vi "Periodic Tasks.vi"(8 "error constant":errorcluster) -> ()   [LabVIEW 2019]
doc: "This VI runs in parallel to other tasks. It can contain as many user-defined periodic loops as you need. These can carry out PID or other sorts of timed response."
uses:
  <vilib>/Rock Robotics/WPI/ThirdParty/Phoenix-LabVIEW/Controls/CTRE_Phoenix_Params.ctl
  <vilib>/Rock Robotics/WPI/ThirdParty/Phoenix-LabVIEW/Motor Controller/Controls/CTRE_Phoenix_MotorControl_ControlMode.ctl
  <vilib>/Rock Robotics/WPI/ThirdParty/Phoenix-LabVIEW/Motor Controller/Controls/CTRE_Phoenix_MotorControl_MotionProfileControlMode.ctl
  <vilib>/Rock Robotics/WPI/Utilities/WPI_GetSetVariantRefNum.vi
  Constants.vi
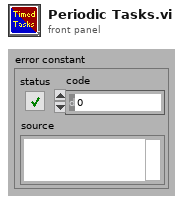
[diagram p1: front panel]
types:
  T1 = enum16{"One_Axis_PercentOutput", "Two_Axis_PercentOutput", "One_Axix_Position", "One_Axis_Position_CustomFeedFwd", "Two_Axis_Position", "One_Axis_Velocity", "One_Axis_Velocity_CustomFeedFwd", "Two_Axis_Velocity", "One_Axis_MotionMagic", "One_Axis_MotionMagic_CustomFeedFwd", "Two_Axis_MotionMagic", "One_Axis_MotionProfile", "One_Axis_MotionProfile_CustomFeedFwd", "Two_Axis_MotionProfile", "Two_Axis_MotionProfile_CustomFeedFwd"}
  T2 = typedef "WPI_MotorControlDeviceRef.ctl" = cluster{"DeviceStatus":errorcluster, "Type":T3, "PWM":cluster{"PWM Channel":T4, "DeadBand":T5}, "CAN":cluster{"Device Number":u8, "SetOutput VI Ref":variant, "GetOutput VI Ref":variant, "Enable VI Ref":variant, "Disable VI Ref":variant, "Data":variant}, "Invert":bool, "DIO PWM":cluster{"PWM \"Enable\" Channel":T4, "DIOChannel":T6, "PWM Rate":dbl}}
  T3 = typedef "WPI_MotorControlType.ctl" = enum16{"PWM", "CAN", "DIO PWM"}
  T4 = typedef "FPGA_DIOPWMChannel.ctl" = enum8{"PWM 0", "PWM 1", "PWM 2", "PWM 3", "PWM 4", "PWM 5", "PWM 6", "PWM 7", "PWM 8", "PWM 9", "PWM MXP 0", "PWM MXP 1", "PWM MXP 2", "PWM MXP 3", "PWM MXP 4", "PWM MXP 5", "PWM MXP 6", "PWM MXP 7", "PWM MXP 8", "PWM MXP 9", "Invalid"}
  T5 = typedef "WPI_PWMDeadband.ctl" = cluster{"Name":string, "maxPositivePwm":i32, "minPositivePwm":i32, "centerPwm":i32, "maxNegativePwm":i32, "minNegativePwm":i32, "angularRange":u16}
  T6 = typedef "FPGA_DIOChannel.ctl" = enum8{"DIO 0", "DIO 1", "DIO 2", "DIO 3", "DIO 4", "DIO 5", "DIO 6", "DIO 7", "DIO 8", "DIO 9", "DIO MXP 0", "DIO MXP 1", "DIO MXP 2", "DIO MXP 3", "DIO MXP 4", "DIO MXP 5", "DIO MXP 6", "DIO MXP 7", "DIO MXP 8", "DIO MXP 9", "DIO MXP 10", "DIO MXP 11", "DIO MXP 12", "DIO MXP 13", "DIO MXP 14", "DIO MXP 15", "SPI Port CS1", "SPI Port CS2", "SPI Port CS3", "SPI Port MISO", "SPI Port MOSI", "Invalid"}
  T7 = typedef "CTRE_PigeonIMU_DeviceRef.ctl" = cluster{"DeviceStatus":errorcluster, "Device Number":u8, "Type":T8, "Device ID":u32, "Handle":u64, "UsageFrame":u32, "Library Path":path}
  T8 = typedef "CTRE_PigeonIMU_ConnectionType.ctl" = u32
  T9 = typedef "WPI_JoystickDevRef.ctl" = cluster{"Device":T10}
  T10 = typedef "WPI_JoystickDeviceEnum.ctl" = enum16{"USB 0", "USB 1", "USB 2", "USB 3", "USB 4", "USB 5"}
  T11 = enum16{"DemandType_Neutral", "DemandType_AuxPID", "DemandType_ArbitraryFeedForward"}
  T12 = enum16{"FollowerType_PercentOutput", "FollowerType_AuxOutput1"}
  T13 = enum16{"One_Axis_PercentOutput", "Two_Axis_PercentOutput", "One_Axix_Position", "One_Axis_Position_CustomFeedFwd", "Two_Axis_Position", "One_Axis_Velocity", "One_Axis_Velocity_CustomFeedFwd", "Two_Axis_Velocity", "One_Axis_MotionMagic", "One_Axis_MotionMagic_CustomFeedFwd", "Two_Axis_MotionMagic", "One_Axis_MotionProfile", "Two_Axis_MotionProfile"}
  T14 = typedef "CTRE_Phoenix_Params.ctl" = u16
  T15 = typedef "CTRE_Phoenix_MotorControl_ControlMode.ctl" = u16
  T16 = typedef "CTRE_Phoenix_MotorControl_MotionProfileControlMode.ctl" = u16
  T17 = typedef "CTRE_Phoenix_MotorControl_BufferedTrajectoryPointStream_DeviceRef.ctl" = cluster{"Handle":u64, "Library Path":path}
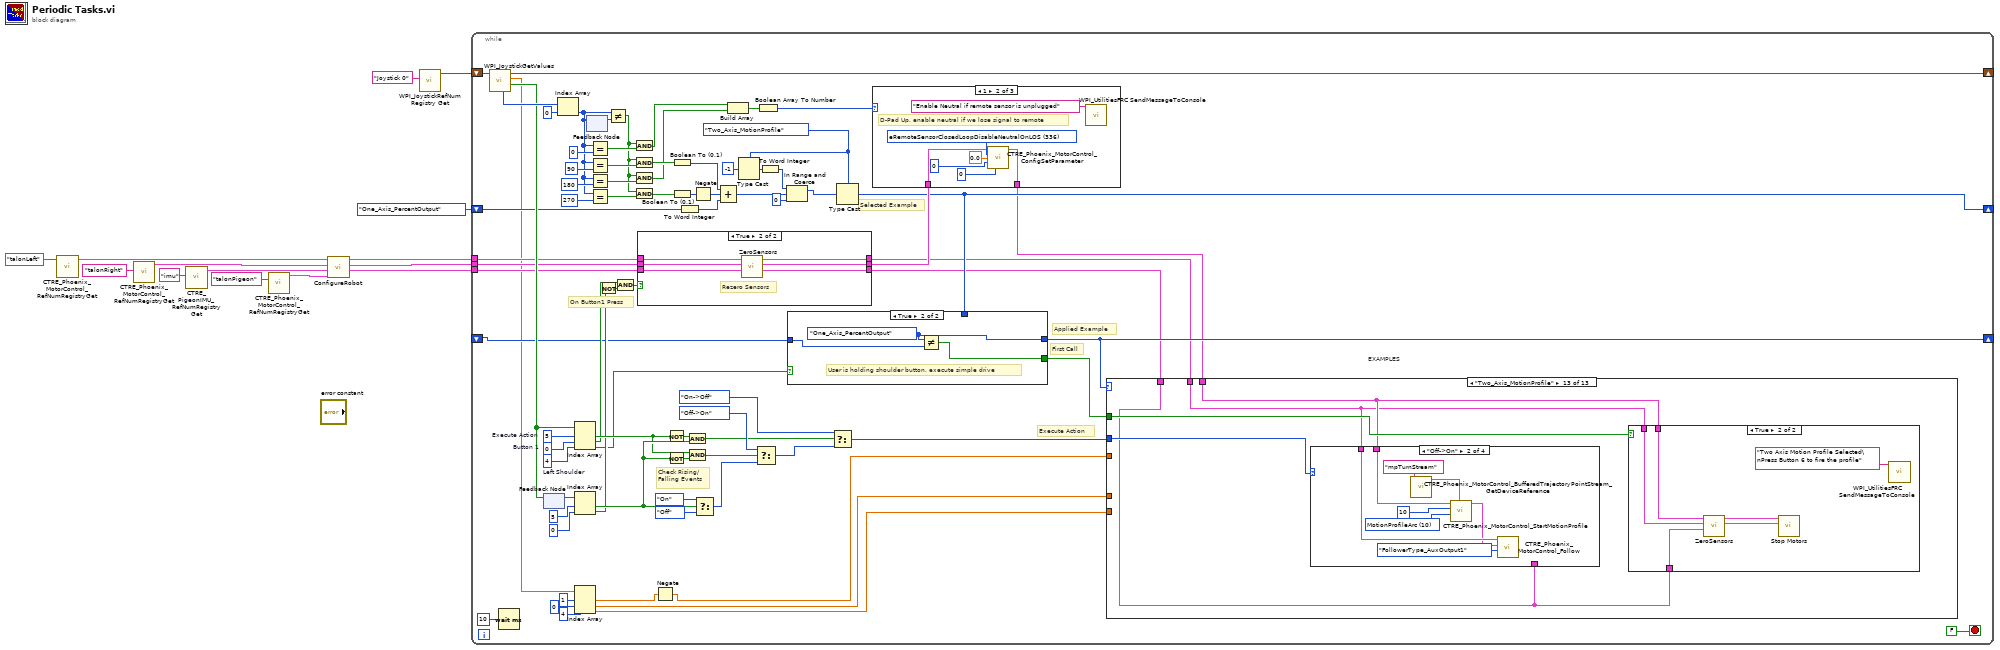
[diagram p0: block diagram]
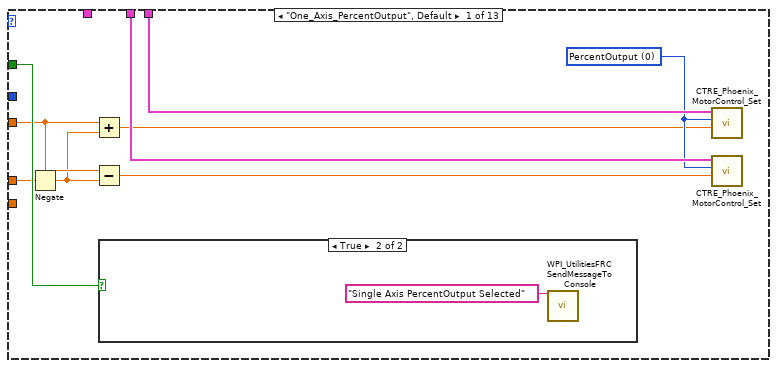
[diagram p2: hidden frame]
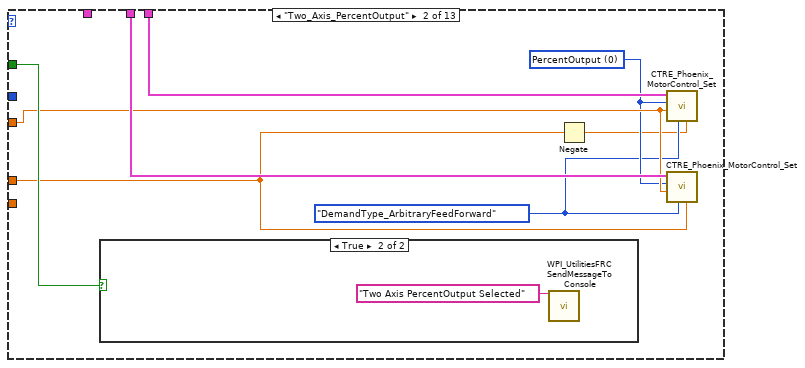
[diagram p4: hidden frame]
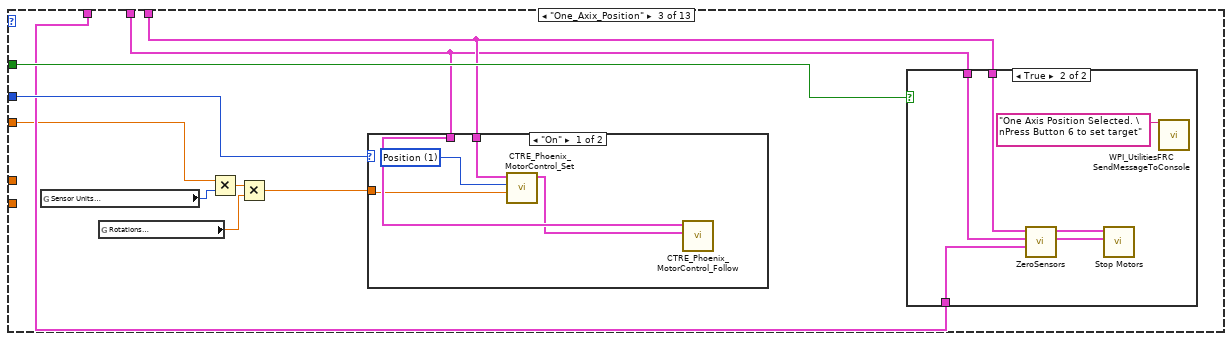
[diagram p6: hidden frame]
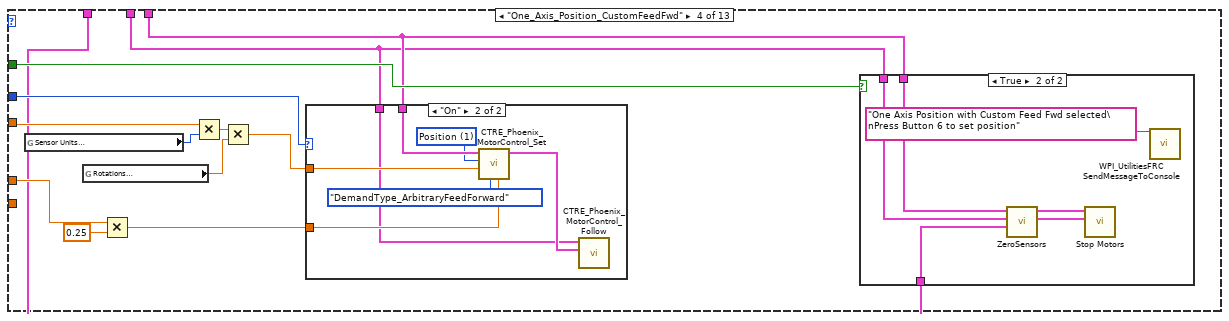
[diagram p9: hidden frame]
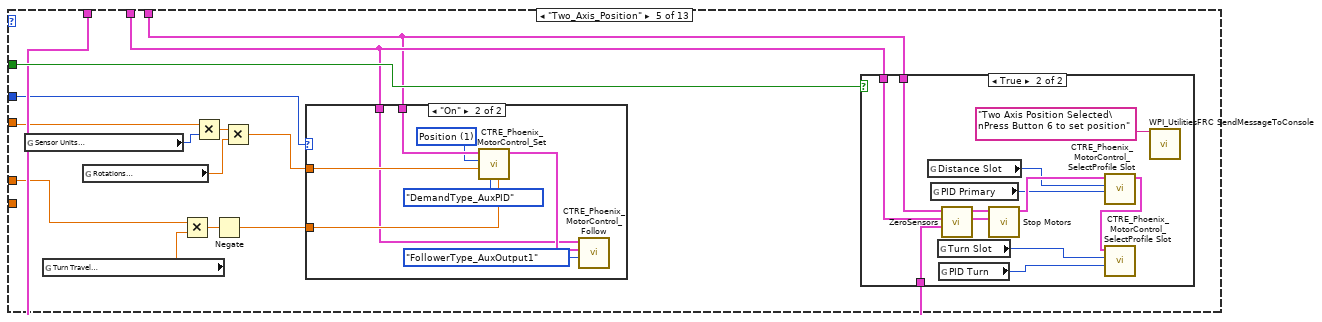
[diagram p12: hidden frame]
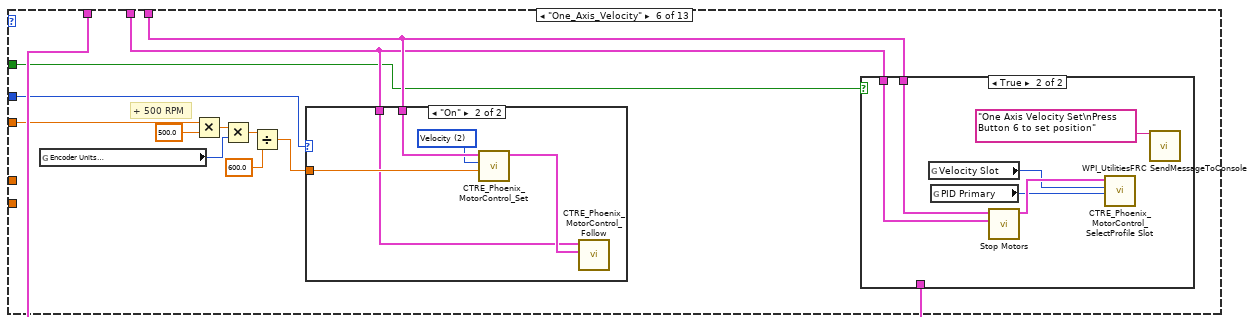
[diagram p15: hidden frame]
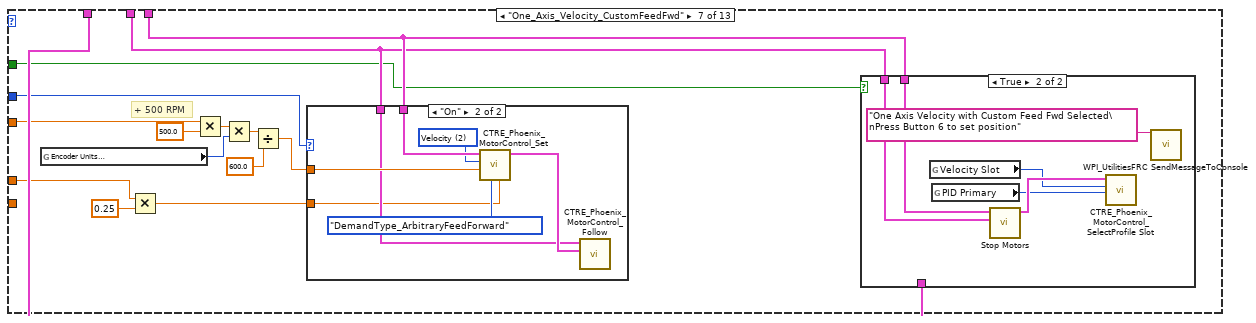
[diagram p18: hidden frame]
diagram:
  n1 = call <vilib>:"CTRE_Phoenix_MotorControl_RefNumRegistryGet.vi"("refnum name"="talonLeft") -> ("PhoenixMotorControlDevRef"=w7:T2)  [unwired: 9 in, 1 out]
  n2 = call <vilib>:"CTRE_Phoenix_MotorControl_RefNumRegistryGet.vi"("refnum name"="talonRight") -> ("PhoenixMotorControlDevRef"=w8:T2)  [unwired: 9 in, 1 out]
  n3 = call <vilib>:"CTRE_PigeonIMU_RefNumRegistryGet.vi"("refnum name"="imu") -> ("PigeonIMUDevRef"=w3:T7)  [unwired: 9 in, 1 out]
  n4 = call <vilib>:"CTRE_Phoenix_MotorControl_RefNumRegistryGet.vi"("refnum name"="talonPigeon") -> ("PhoenixMotorControlDevRef"=w2:T2)  [unwired: 9 in, 1 out]
  n5 = call "ConfigureRobot.vi"("Pigeon Talon"=w2, "Pigeon"=w3, "Right Side"=w8, "Left Side"=w7) -> ("Pigeon 2"=w4:T7, "Right Side 2"=w1:T2, "Left Side 2"=w5:T2)  [unwired: 5 in]
  n6 = call <vilib>:"WPI_JoystickRefNum Registry Get.vi"("refnum name"="Joystick 0") -> ("JoystickDevRef"=w13:T9)  [unwired: 1 in, 9 out]
  n7 = while {
    shift-right: [w90] -> _
    shift-left: w13 -> [w91]
    shift-right: [w40] -> _
    shift-left: T1."One_Axis_PercentOutput" -> [w39]
    tunnel: w5 -> [w54]
    tunnel: w1 -> [w53]
    tunnel: w4 -> [w52]
    shift-right: [w41] -> _
    shift-left: _ -> [w42]
    stop <- FALSE stop-if-true
    w33 = T13."Two_Axis_MotionProfile"
    w44 = 4  # Left Shoulder
    w50 = 0  # Button 1
    w68 = 5  # Execute Action
    # "Execute Action"
    # "Check Rising/\nFalling Events"
    # "First Call"
    # "Applied Example"
    # "On Button1 Press"
    # "Selected Example"
    n8 = call <vilib>:"WPI_JoystickGetValues.vi"("JoystickDevRef"=w91) -> ("Buttons"=w70:bool[], "Axes"=w28:dbl[], "JoystickDevRef"=w90:T9, "POVs"=w89:i16[])  [unwired: 6 in, 1 out]
    n9 = Wait (ms)(milliseconds to wait=u32 10) -> ()  [unwired: 1 out]
    n10 = feedback #1() -> (w69:bool[])  [unwired: 1 in]
    n11 = feedback-in #1(w70) -> ()
    n12 = Index Array(array=w89, index=0) -> (element=w82:i16)
    n13 = Index Array(array=w70, index #1=w68, index #2=w50, index #3=w44) -> (element #1=w61:bool, element #2=w47:bool, element #3=w43:bool)
    n14 = Index Array(array=w69, index #1=5 ("index"), index #2=0 ("index")) -> (element #1=w62:bool, element #2=w45:bool)
    n15 = Index Array(array=w28, index #1=1 ("index"), index #2=0 ("index"), index #3=4 ("index")) -> (element #1=w17:dbl, element #2=w25:dbl, element #3=w18:dbl)
    n16 = feedback #2() -> (w83:i16)  [unwired: 1 in]
    n17 = feedback-in #2(w82) -> ()
    n18 = Equal?(x=w82, y=i16 0) -> (x = y?=w81:bool)
    n19 = Equal?(x=w82, y=i16 90) -> (x = y?=w80:bool)
    n20 = Equal?(x=w82, y=i16 180) -> (x = y?=w79:bool)
    n21 = Equal?(x=w82, y=i16 270) -> (x = y?=w78:bool)
    n22 = Not(x=w45) -> (.not. x?=w46:bool)
    n23 = Not Equal?(x=w82, y=w83) -> (x != y?=w77:bool)
    n24 = And(x=w47, y=w46) -> (x .and. y?=w48:bool)
    n25 = And(x=w77, y=w81) -> (x .and. y?=w72:bool)
    n26 = And(x=w77, y=w80) -> (x .and. y?=w75:bool)
    n27 = And(x=w77, y=w79) -> (x .and. y?=w71:bool)
    n28 = And(x=w77, y=w78) -> (x .and. y?=w76:bool)
    n29 = case shown="True" w48 {
      tunnel: w54 -> [w422 w424]
      tunnel: w53 -> [w423 w425]
      tunnel: w52 -> [w421 w426]
      tunnel: [w423 w428] -> w51
      tunnel: [w422 w429] -> w24
      tunnel: [w421 w427] -> w15
      frame False {
        # "Do Nothing"
      }
      frame True {
        # "Rezero Sensors"
        n30 = call "ZeroSensors.vi"("Pigeon"=w426, "Talon 2"=w425, "Talon 1"=w424) -> ("Pigeon"=w427:T7, "Talon 2"=w428:T2, "Talon 1"=w429:T2)  [unwired: 6 in]
      }
    }
    n31 = Negate(x=w17) -> (-x=w16:dbl)
    n32 = Not(x=w61) -> (.not. x?=w63:bool)
    n33 = Not(x=w62) -> (.not. x?=w64:bool)
    n34 = Boolean To (0,1)(Boolean=w75) -> (0, 1=w22:i16)
    n35 = Boolean To (0,1)(Boolean=w76) -> (0, 1=w20:i16)
    n36 = To Word Integer(number=w39) -> (16bit integer=w38:i16)
    n37 = And(x=w63, y=w62) -> (x .and. y?=w55:bool)
    n38 = And(x=w61, y=w64) -> (x .and. y?=w56:bool)
    n39 = Negate(x=w20) -> (-x=w21:i16)
    n40 = Select(t=enum16{"Off->On", "On->Off", "On", "Off"}."On", s=w62, f=enum16{"Off->On", "On->Off", "On", "Off"}."Off") -> (s? t:f=w60:enum16{"Off->On", "On->Off", "On", "Off"})
    n41 = Compound Arithmetic op=ADD(w22, w21, w38) -> (w37:i16)
    n42 = Build Array(w72, w71) -> (w73:bool[])
    n43 = Type Cast(type=w33, x=i16 -1 ("lower limit")) -> (*(type *) &x=w31:T13)
    n44 = Select(t=enum16{"Off->On", "On->Off", "On", "Off"}."Off->On", s=w56, f=w60) -> (s? t:f=w59:enum16{"Off->On", "On->Off", "On", "Off"})
    n45 = Boolean Array To Number(Boolean array=w73) -> (number=w74:u32)
    n46 = To Word Integer(number=w31) -> (16bit integer=w32:i16)
    n47 = In Range and Coerce(upper limit=w32, x=w37, lower limit=i16 0) -> (coerced(x)=w35:i16)  [unwired: 1 out]
    n48 = Select(t=enum16{"Off->On", "On->Off", "On", "Off"}."On->Off", s=w55, f=w59) -> (s? t:f=w29:enum16{"Off->On", "On->Off", "On", "Off"})
    n49 = Type Cast(type=w33, x=w35) -> (*(type *) &x=w40:T13)
    n50 = case shown="True" w43 {
      tunnel: w42 -> [w415 w420]
      tunnel: [w417 w419] -> w30
      tunnel: [w416 w418] -> w41
      tunnel: w40 -> [w416 _]
      frame False {
        # "User is not holding shoulder button, use applied example"
        n51 = Not Equal?(x=w416, y=w415) -> (x != y?=w417:bool)
      }
      frame True {
        w418 = T13."One_Axis_PercentOutput"
        # "User is holding shoulder button, execute simple drive"
        n52 = Not Equal?(x=w418, y=w420) -> (x != y?=w419:bool)
      }
    }
    n53 = case shown="1" w74 {
      tunnel: w51 -> [w430 w432 w444]
      tunnel: [w430 w433 w443] -> w23
      frame 0, Default {
        # "Nothing Pressed"
      }
      frame 1 {
        w437 = T14 336 items=["eOnBoot_BrakeMode"=31, "eQuadFilterEn"=91, "eQuadIdxPolarity"=108, "eClearPositionOnIdx"=100, "eMotionProfileHasUnderrunErr"=119, "eMotionProfileTrajectoryPointDurationMs"=120, "eClearPosOnLimitF"=144, "eClearPosOnLimitR"=145, "eStatusFramePeriod"=300, "eOpenLoopRamp"=301, "eClosedLoopRamp"=302, "eNeutralDeadband"=303, "ePeakPosOutput"=305, "eNominalPosOutput"=306, "ePeakNegOutput"=307, "eNominalNegOutput"=308, "eProfileParamSlot_P"=310, "eProfileParamSlot_I"=311, "eProfileParamSlot_D"=312, "eProfileParamSlot_F"=313, "eProfileParamSlot_IZone"=314, "eProfileParamSlot_AllowableErr"=315, "eProfileParamSlot_MaxIAccum"=316, "eClearPositionOnLimitF"=320, "eClearPositionOnLimitR"=321, "eClearPositionOnQuadIdx"=322, "eSampleVelocityPeriod"=325, "eSampleVelocityWindow"=326, "eFeedbackSensorType"=330, "eSelectedSensorPosition"=331, "eFeedbackNotContinuous"=332, "eRemoteSensorSource"=333, "eRemoteSensorDeviceID"=334, "eSensorTerm"=335, "eRemoteSensorClosedLoopDisableNeutralOnLOS"=336, "eForwardSoftLimitThreshold"=340, "eReverseSoftLimitThreshold"=341, "eForwardSoftLimitEnable"=342, "eReverseSoftLimitEnable"=343, "eNominalBatteryVoltage"=350, "eBatterVoltageFilterSize"=351, "eContinuousCurrentLimitAmps"=360, "eContinuousCurrentLimitMs"=361, "ePeakCurrentLimitAmps"=362, "eClosedLoopIAccum"=370, "eCustomParam"=380, "eStickyFaults"=390, "eAnalogPosition"=400, "eQuadraturePosition"=401, "ePulseWidthPosition"=402, "eMotMag_Accel"=410, "eMotMag_VelCruise"=411, "eLimitSwitchSource"=421, "eLimitSwitchNormClosedAndDis"=422, "eLimitSwitchDisabledNeutralOnLOS"=423, "eLimitSwitchRemoteDevID"=424] ("Parameter")
        # "D-Pad Up, enable neutral if we lose signal to remote"
        n54 = call <vilib>:"CTRE_Phoenix_MotorControl_ConfigSetParameter.vi"("PhoenixMotorControlDevRef"=w432, "Parameter"=w437, "value"=0.0, "subValue"=u8 0, "ordinal"=0) -> ("PhoenixMotorControlDevRef"=w433:T2)  [unwired: 9 in, 1 out]
        n55 = call <vilib>:"WPI_UtilitiesFRC SendMessageToConsole.vi"("Message"="Enable Neutral if remote sensor is unplugged") -> ()  [unwired: 14 in, 1 out]
      }
      frame 2 {
        w442 = T14 336 items=["eOnBoot_BrakeMode"=31, "eQuadFilterEn"=91, "eQuadIdxPolarity"=108, "eClearPositionOnIdx"=100, "eMotionProfileHasUnderrunErr"=119, "eMotionProfileTrajectoryPointDurationMs"=120, "eClearPosOnLimitF"=144, "eClearPosOnLimitR"=145, "eStatusFramePeriod"=300, "eOpenLoopRamp"=301, "eClosedLoopRamp"=302, "eNeutralDeadband"=303, "ePeakPosOutput"=305, "eNominalPosOutput"=306, "ePeakNegOutput"=307, "eNominalNegOutput"=308, "eProfileParamSlot_P"=310, "eProfileParamSlot_I"=311, "eProfileParamSlot_D"=312, "eProfileParamSlot_F"=313, "eProfileParamSlot_IZone"=314, "eProfileParamSlot_AllowableErr"=315, "eProfileParamSlot_MaxIAccum"=316, "eClearPositionOnLimitF"=320, "eClearPositionOnLimitR"=321, "eClearPositionOnQuadIdx"=322, "eSampleVelocityPeriod"=325, "eSampleVelocityWindow"=326, "eFeedbackSensorType"=330, "eSelectedSensorPosition"=331, "eFeedbackNotContinuous"=332, "eRemoteSensorSource"=333, "eRemoteSensorDeviceID"=334, "eSensorTerm"=335, "eRemoteSensorClosedLoopDisableNeutralOnLOS"=336, "eForwardSoftLimitThreshold"=340, "eReverseSoftLimitThreshold"=341, "eForwardSoftLimitEnable"=342, "eReverseSoftLimitEnable"=343, "eNominalBatteryVoltage"=350, "eBatterVoltageFilterSize"=351, "eContinuousCurrentLimitAmps"=360, "eContinuousCurrentLimitMs"=361, "ePeakCurrentLimitAmps"=362, "eClosedLoopIAccum"=370, "eCustomParam"=380, "eStickyFaults"=390, "eAnalogPosition"=400, "eQuadraturePosition"=401, "ePulseWidthPosition"=402, "eMotMag_Accel"=410, "eMotMag_VelCruise"=411, "eLimitSwitchSource"=421, "eLimitSwitchNormClosedAndDis"=422, "eLimitSwitchDisabledNeutralOnLOS"=423, "eLimitSwitchRemoteDevID"=424] ("Parameter")
        # "D-Pad Up, disable neutral if we lose signal to remote"
        n56 = call <vilib>:"CTRE_Phoenix_MotorControl_ConfigSetParameter.vi"("PhoenixMotorControlDevRef"=w444, "Parameter"=w442, "value"=1.0, "subValue"=u8 0, "ordinal"=0) -> ("PhoenixMotorControlDevRef"=w443:T2)  [unwired: 9 in, 1 out]
        n57 = call <vilib>:"WPI_UtilitiesFRC SendMessageToConsole.vi"("Message"="Disable Neutral if remote sensor is unplugged") -> ()  [unwired: 14 in, 1 out]
      }
    }
    n58 = case "EXAMPLES" shown="\"Two_Axis_MotionProfile\"" w41 {
      tunnel: w30 -> [w100 w111 w122 w146 w169 w201 w222 w254 w282 w308 w328 w364 w392]
      tunnel: w29 -> [_ _ w121 w145 w165 w200 w221 w253 w281 w309 w334 w363 w391]
      tunnel: w16 -> [w98 w108 w113 w141 w164 w199 w220 w252 w280 w310 w333 _ _]
      tunnel: w25 -> [w95 w105 _ w140 w163 _ w219 w251 _ w304 w332 _ _]
      tunnel: w24 -> [w101 w109 w115 w135 w167 w203 w224 w249 w283 w306 w330 w365 w389]
      tunnel: w23 -> [w102 w110 w116 w136 w166 w204 w225 w248 w285 w305 w329 w366 w390]
      tunnel: w15 -> [_ _ w114 w134 w168 w202 w223 w250 w284 w307 w331 w362 w388]
      tunnel: w18 -> [_ _ _ _ _ _ _ _ _ _ _ _ _]
      frame "One_Axis_PercentOutput", Default {
        w99 = T15 0 items=["PercentOutput"=0, "Position"=1, "Velocity"=2, "Current"=3, "Follower"=5, "MotionProfile"=6, "MotionMagic"=7, "MotionMagicArc"=8, "MotionProfileArc"=10, "Disabled"=15] ("Control Mode")
        n59 = Negate(x=w95) -> (-x=w94:dbl)
        n60 = Add(x=w98, y=w94) -> (x+y=w96:dbl)
        n61 = Subtract(x=w98, y=w94) -> (x-y=w97:dbl)
        n62 = case shown="True" w100 {
          frame False {
          }
          frame True {
            n63 = call <vilib>:"WPI_UtilitiesFRC SendMessageToConsole.vi"("Message"="Single Axis PercentOutput Selected") -> ()  [unwired: 14 in, 1 out]
          }
        }
        n64 = call <vilib>:"CTRE_Phoenix_MotorControl_Set.vi"("Output"=w96, "Control Mode"=w99, "PhoenixMotorControlDevRef"=w102) -> ()  [unwired: 7 in, 2 out]
        n65 = call <vilib>:"CTRE_Phoenix_MotorControl_Set.vi"("Output"=w97, "Control Mode"=w99, "PhoenixMotorControlDevRef"=w101) -> ()  [unwired: 7 in, 2 out]
      }
      frame "Two_Axis_PercentOutput" {
        w106 = T11."DemandType_ArbitraryFeedForward" ("DemandType")
        w107 = T15 0 items=["PercentOutput"=0, "Position"=1, "Velocity"=2, "Current"=3, "Follower"=5, "MotionProfile"=6, "MotionMagic"=7, "MotionMagicArc"=8, "MotionProfileArc"=10, "Disabled"=15] ("Control Mode")
        n66 = case shown="True" w111 {
          frame False {
          }
          frame True {
            n67 = call <vilib>:"WPI_UtilitiesFRC SendMessageToConsole.vi"("Message"="Two Axis PercentOutput Selected") -> ()  [unwired: 14 in, 1 out]
          }
        }
        n68 = Negate(x=w105) -> (-x=w104:dbl)
        n69 = call <vilib>:"CTRE_Phoenix_MotorControl_Set.vi"("Demand1"=w104, "DemandType"=w106, "Output"=w108, "Control Mode"=w107, "PhoenixMotorControlDevRef"=w110) -> ()  [unwired: 5 in, 2 out]
        n70 = call <vilib>:"CTRE_Phoenix_MotorControl_Set.vi"("Demand1"=w105, "DemandType"=w106, "Output"=w108, "Control Mode"=w107, "PhoenixMotorControlDevRef"=w109) -> ()  [unwired: 5 in, 2 out]
      }
      frame "One_Axix_Position" {
        n71 = global read "Constants.vi" "Sensor Units\nPer Rotation"() -> (w119:i32)
        n72 = global read "Constants.vi" "Rotations\nTo Travel"() -> (w118:dbl)
        n73 = Multiply(x=w113, y=w119) -> (x*y=w120:dbl)
        n74 = Multiply(x=w120, y=w118) -> (x*y=w117:dbl)
        n75 = case shown="\"On\"" w121 {
          tunnel: w117 -> [w123 _]
          tunnel: w116 -> [w127 _]
          tunnel: w115 -> [w125 _]
          frame "On" {
            w126 = T15 1 items=["PercentOutput"=0, "Position"=1, "Velocity"=2, "Current"=3, "Follower"=5, "MotionProfile"=6, "MotionMagic"=7, "MotionProfileArc"=10, "Disabled"=15] ("Control Mode")
            n76 = call <vilib>:"CTRE_Phoenix_MotorControl_Set.vi"("Output"=w123, "Control Mode"=w126, "PhoenixMotorControlDevRef"=w127) -> ("PhoenixMotorControlDevRef"=w124:T2)  [unwired: 7 in, 1 out]
            n77 = call <vilib>:"CTRE_Phoenix_MotorControl_Follow.vi"("Master Controller to Follow"=w124, "PhoenixMotorControlDevRef"=w125) -> ()  [unwired: 8 in, 2 out]
          }
          frame Default {
          }
        }
        n78 = case shown="True" w122 {
          tunnel: w116 -> [_ w132]
          tunnel: w115 -> [_ w131]
          tunnel: w114 -> [_ w130]
          frame False {
          }
          frame True {
            n79 = call "ZeroSensors.vi"("Pigeon"=w130, "Talon 2"=w131, "Talon 1"=w132) -> ("Talon 2"=w128:T2, "Talon 1"=w129:T2)  [unwired: 6 in, 1 out]
            n80 = call "Stop Motors.vi"("Talon SRX 2"=w128, "Talon SRX 1"=w129) -> ()  [unwired: 8 in, 2 out]
            n81 = call <vilib>:"WPI_UtilitiesFRC SendMessageToConsole.vi"("Message"="One Axis Position Selected. \nPress Button 6 to set target") -> ()  [unwired: 14 in, 1 out]
          }
        }
      }
      frame "One_Axis_Position_CustomFeedFwd" {
        n82 = global read "Constants.vi" "Sensor Units\nPer Rotation"() -> (w143:i32)
        n83 = global read "Constants.vi" "Rotations\nTo Travel"() -> (w142:dbl)
        n84 = Multiply(x=w140, y=0.25) -> (x*y=w137:dbl)
        n85 = Multiply(x=w141, y=w143) -> (x*y=w144:dbl)
        n86 = Multiply(x=w144, y=w142) -> (x*y=w138:dbl)
        n87 = case shown="\"On\"" w145 {
          tunnel: w136 -> [_ w153]
          tunnel: w135 -> [_ w147]
          tunnel: w137 -> [_ w149]
          tunnel: w138 -> [_ w151]
          frame Default {
          }
          frame "On" {
            w152 = T15 1 items=["PercentOutput"=0, "Position"=1, "Velocity"=2, "Current"=3, "Follower"=5, "MotionProfile"=6, "MotionMagic"=7, "MotionProfileArc"=10, "Disabled"=15] ("Control Mode")
            n88 = call <vilib>:"CTRE_Phoenix_MotorControl_Set.vi"("Demand1"=w149, "DemandType"=T11."DemandType_ArbitraryFeedForward", "Output"=w151, "Control Mode"=w152, "PhoenixMotorControlDevRef"=w153) -> ("PhoenixMotorControlDevRef"=w148:T2)  [unwired: 5 in, 1 out]
            n89 = call <vilib>:"CTRE_Phoenix_MotorControl_Follow.vi"("Master Controller to Follow"=w148, "PhoenixMotorControlDevRef"=w147) -> ()  [unwired: 8 in, 2 out]
          }
        }
        n90 = case shown="True" w146 {
          tunnel: w136 -> [_ w156]
          tunnel: w135 -> [_ w155]
          tunnel: w134 -> [_ w154]
          frame False {
          }
          frame True {
            n91 = call "ZeroSensors.vi"("Pigeon"=w154, "Talon 2"=w155, "Talon 1"=w156) -> ("Talon 2"=w157:T2, "Talon 1"=w158:T2)  [unwired: 6 in, 1 out]
            n92 = call "Stop Motors.vi"("Talon SRX 2"=w157, "Talon SRX 1"=w158) -> ()  [unwired: 8 in, 2 out]
            n93 = call <vilib>:"WPI_UtilitiesFRC SendMessageToConsole.vi"("Message"="One Axis Position with Custom Feed Fwd selected\nPress Button 6 to set position") -> ()  [unwired: 14 in, 1 out]
          }
        }
      }
      frame "Two_Axis_Position" {
        n94 = global read "Constants.vi" "Sensor Units\nPer Rotation"() -> (w172:i32)
        n95 = global read "Constants.vi" "Turn Travel\nUnits Per Rotation"() -> (w162:dbl)
        n96 = global read "Constants.vi" "Rotations\nTo Travel"() -> (w171:dbl)
        n97 = Multiply(x=w163, y=w162) -> (x*y=w161:dbl)
        n98 = Multiply(x=w164, y=w172) -> (x*y=w173:dbl)
        n99 = Negate(x=w161) -> (-x=w160:dbl)
        n100 = Multiply(x=w173, y=w171) -> (x*y=w170:dbl)
        n101 = case shown="\"On\"" w165 {
          tunnel: w166 -> [_ w181]
          tunnel: w167 -> [_ w175]
          tunnel: w160 -> [_ w177]
          tunnel: w170 -> [_ w179]
          frame Default {
          }
          frame "On" {
            w180 = T15 1 items=["PercentOutput"=0, "Position"=1, "Velocity"=2, "Current"=3, "Follower"=5, "MotionProfile"=6, "MotionMagic"=7, "MotionProfileArc"=10, "Disabled"=15] ("Control Mode")
            n102 = call <vilib>:"CTRE_Phoenix_MotorControl_Set.vi"("Demand1"=w177, "DemandType"=T11."DemandType_AuxPID", "Output"=w179, "Control Mode"=w180, "PhoenixMotorControlDevRef"=w181) -> ("PhoenixMotorControlDevRef"=w176:T2)  [unwired: 5 in, 1 out]
            n103 = call <vilib>:"CTRE_Phoenix_MotorControl_Follow.vi"("FollowerType"=T12."FollowerType_AuxOutput1", "Master Controller to Follow"=w176, "PhoenixMotorControlDevRef"=w175) -> ()  [unwired: 7 in, 2 out]
          }
        }
        n104 = case shown="True" w169 {
          tunnel: w166 -> [_ w190]
          tunnel: w167 -> [_ w189]
          tunnel: w168 -> [_ w188]
          frame False {
          }
          frame True {
            n105 = global read "Constants.vi" "Distance Slot"() -> (w185:i32)
            n106 = global read "Constants.vi" "PID Primary"() -> (w186:i32)
            n107 = global read "Constants.vi" "Turn Slot"() -> (w184:i32)
            n108 = global read "Constants.vi" "PID Turn"() -> (w183:i32)
            n109 = call "ZeroSensors.vi"("Pigeon"=w188, "Talon 2"=w189, "Talon 1"=w190) -> ("Talon 2"=w191:T2, "Talon 1"=w192:T2)  [unwired: 6 in, 1 out]
            n110 = call "Stop Motors.vi"("Talon SRX 2"=w191, "Talon SRX 1"=w192) -> ("Talon SRX 1"=w187:T2)  [unwired: 8 in, 1 out]
            n111 = call <vilib>:"CTRE_Phoenix_MotorControl_SelectProfile Slot.vi"("pidLoopIdx"=w186, "slotIdx"=w185, "PhoenixMotorControlDevRef"=w187) -> ("PhoenixMotorControlDevRef"=w182:T2)  [unwired: 7 in, 1 out]
            n112 = call <vilib>:"CTRE_Phoenix_MotorControl_SelectProfile Slot.vi"("pidLoopIdx"=w183, "slotIdx"=w184, "PhoenixMotorControlDevRef"=w182) -> ()  [unwired: 7 in, 2 out]
            n113 = call <vilib>:"WPI_UtilitiesFRC SendMessageToConsole.vi"("Message"="Two Axis Position Selected\nPress Button 6 to set position") -> ()  [unwired: 14 in, 1 out]
          }
        }
      }
      frame "One_Axis_Velocity" {
        # "+ 500 RPM"
        n114 = global read "Constants.vi" "Encoder Units\nPer Rotation"() -> (w197:i32)
        n115 = Multiply(x=w199, y=500.0) -> (x*y=w205:dbl)
        n116 = Multiply(x=w205, y=w197) -> (x*y=w196:dbl)
        n117 = Divide(x=w196, y=600.0) -> (x/y=w195:dbl)
        n118 = case shown="\"On\"" w200 {
          tunnel: w204 -> [_ w210]
          tunnel: w203 -> [_ w206]
          tunnel: w195 -> [_ w208]
          frame Default {
          }
          frame "On" {
            w209 = T15 2 items=["PercentOutput"=0, "Position"=1, "Velocity"=2, "Current"=3, "Follower"=5, "MotionProfile"=6, "MotionMagic"=7, "MotionProfileArc"=10, "Disabled"=15] ("Control Mode")
            n119 = call <vilib>:"CTRE_Phoenix_MotorControl_Set.vi"("Output"=w208, "Control Mode"=w209, "PhoenixMotorControlDevRef"=w210) -> ("PhoenixMotorControlDevRef"=w207:T2)  [unwired: 7 in, 1 out]
            n120 = call <vilib>:"CTRE_Phoenix_MotorControl_Follow.vi"("Master Controller to Follow"=w207, "PhoenixMotorControlDevRef"=w206) -> ()  [unwired: 8 in, 2 out]
          }
        }
        n121 = case shown="True" w201 {
          tunnel: w204 -> [_ w212]
          tunnel: w203 -> [_ w211]
          tunnel: w202 -> [_ _]
          frame False {
          }
          frame True {
            n122 = global read "Constants.vi" "Velocity Slot"() -> (w213:i32)
            n123 = global read "Constants.vi" "PID Primary"() -> (w214:i32)
            n124 = call "Stop Motors.vi"("Talon SRX 2"=w211, "Talon SRX 1"=w212) -> ("Talon SRX 1"=w215:T2)  [unwired: 8 in, 1 out]
            n125 = call <vilib>:"CTRE_Phoenix_MotorControl_SelectProfile Slot.vi"("pidLoopIdx"=w214, "slotIdx"=w213, "PhoenixMotorControlDevRef"=w215) -> ()  [unwired: 7 in, 2 out]
            n126 = call <vilib>:"WPI_UtilitiesFRC SendMessageToConsole.vi"("Message"="One Axis Velocity Set\nPress Button 6 to set position") -> ()  [unwired: 14 in, 1 out]
          }
        }
      }
      frame "One_Axis_Velocity_CustomFeedFwd" {
        # "+ 500 RPM"
        n127 = global read "Constants.vi" "Encoder Units\nPer Rotation"() -> (w229:i32)
        n128 = Multiply(x=w219, y=0.25) -> (x*y=w217:dbl)
        n129 = Multiply(x=w220, y=500.0) -> (x*y=w231:dbl)
        n130 = Multiply(x=w231, y=w229) -> (x*y=w228:dbl)
        n131 = Divide(x=w228, y=600.0) -> (x/y=w227:dbl)
        n132 = case shown="\"On\"" w221 {
          tunnel: w225 -> [_ w238]
          tunnel: w224 -> [_ w234]
          tunnel: w227 -> [_ w236]
          tunnel: w217 -> [_ w232]
          frame Default {
          }
          frame "On" {
            w237 = T15 2 items=["PercentOutput"=0, "Position"=1, "Velocity"=2, "Current"=3, "Follower"=5, "MotionProfile"=6, "MotionMagic"=7, "MotionProfileArc"=10, "Disabled"=15] ("Control Mode")
            n133 = call <vilib>:"CTRE_Phoenix_MotorControl_Set.vi"("Demand1"=w232, "DemandType"=T11."DemandType_ArbitraryFeedForward", "Output"=w236, "Control Mode"=w237, "PhoenixMotorControlDevRef"=w238) -> ("PhoenixMotorControlDevRef"=w235:T2)  [unwired: 5 in, 1 out]
            n134 = call <vilib>:"CTRE_Phoenix_MotorControl_Follow.vi"("Master Controller to Follow"=w235, "PhoenixMotorControlDevRef"=w234) -> ()  [unwired: 8 in, 2 out]
          }
        }
        n135 = case shown="True" w222 {
          tunnel: w225 -> [_ w240]
          tunnel: w224 -> [_ w239]
          tunnel: w223 -> [_ _]
          frame False {
          }
          frame True {
            n136 = global read "Constants.vi" "Velocity Slot"() -> (w241:i32)
            n137 = global read "Constants.vi" "PID Primary"() -> (w242:i32)
            n138 = call "Stop Motors.vi"("Talon SRX 2"=w239, "Talon SRX 1"=w240) -> ("Talon SRX 1"=w243:T2)  [unwired: 8 in, 1 out]
            n139 = call <vilib>:"CTRE_Phoenix_MotorControl_SelectProfile Slot.vi"("pidLoopIdx"=w242, "slotIdx"=w241, "PhoenixMotorControlDevRef"=w243) -> ()  [unwired: 7 in, 2 out]
            n140 = call <vilib>:"WPI_UtilitiesFRC SendMessageToConsole.vi"("Message"="One Axis Velocity with Custom Feed Fwd Selected\nPress Button 6 to set position") -> ()  [unwired: 14 in, 1 out]
          }
        }
      }
      frame "Two_Axis_Velocity" {
        # "+ 500 RPM"
        n141 = global read "Constants.vi" "Turn Travel\nUnits Per Rotation"() -> (w247:dbl)
        n142 = global read "Constants.vi" "Encoder Units\nPer Rotation"() -> (w258:i32)
        n143 = Multiply(x=w251, y=w247) -> (x*y=w246:dbl)
        n144 = Multiply(x=w252, y=500.0) -> (x*y=w260:dbl)
        n145 = Multiply(x=w260, y=w258) -> (x*y=w257:dbl)
        n146 = Negate(x=w246) -> (-x=w245:dbl)
        n147 = Divide(x=w257, y=600.0) -> (x/y=w256:dbl)
        n148 = case shown="\"On\"" w253 {
          tunnel: w248 -> [_ w268]
          tunnel: w249 -> [_ w264]
          tunnel: w256 -> [_ w266]
          tunnel: w245 -> [_ w262]
          frame Default {
          }
          frame "On" {
            w267 = T15 2 items=["PercentOutput"=0, "Position"=1, "Velocity"=2, "Current"=3, "Follower"=5, "MotionProfile"=6, "MotionMagic"=7, "MotionProfileArc"=10, "Disabled"=15] ("Control Mode")
            n149 = call <vilib>:"CTRE_Phoenix_MotorControl_Set.vi"("Demand1"=w262, "DemandType"=T11."DemandType_AuxPID", "Output"=w266, "Control Mode"=w267, "PhoenixMotorControlDevRef"=w268) -> ("PhoenixMotorControlDevRef"=w265:T2)  [unwired: 5 in, 1 out]
            n150 = call <vilib>:"CTRE_Phoenix_MotorControl_Follow.vi"("FollowerType"=T12."FollowerType_AuxOutput1", "Master Controller to Follow"=w265, "PhoenixMotorControlDevRef"=w264) -> ()  [unwired: 7 in, 2 out]
          }
        }
        n151 = case shown="True" w254 {
          tunnel: w248 -> [_ w273]
          tunnel: w249 -> [_ w272]
          tunnel: w250 -> [_ _]
          frame False {
          }
          frame True {
            n152 = global read "Constants.vi" "Velocity Slot"() -> (w274:i32)
            n153 = global read "Constants.vi" "PID Primary"() -> (w275:i32)
            n154 = global read "Constants.vi" "Turn Slot"() -> (w271:i32)
            n155 = global read "Constants.vi" "PID Turn"() -> (w269:i32)
            n156 = call "Stop Motors.vi"("Talon SRX 2"=w272, "Talon SRX 1"=w273) -> ("Talon SRX 1"=w276:T2)  [unwired: 8 in, 1 out]
            n157 = call <vilib>:"CTRE_Phoenix_MotorControl_SelectProfile Slot.vi"("pidLoopIdx"=w275, "slotIdx"=w274, "PhoenixMotorControlDevRef"=w276) -> ("PhoenixMotorControlDevRef"=w270:T2)  [unwired: 7 in, 1 out]
            n158 = call <vilib>:"CTRE_Phoenix_MotorControl_SelectProfile Slot.vi"("pidLoopIdx"=w269, "slotIdx"=w271, "PhoenixMotorControlDevRef"=w270) -> ()  [unwired: 7 in, 2 out]
            n159 = call <vilib>:"WPI_UtilitiesFRC SendMessageToConsole.vi"("Message"="Two Axis Velocity\nPress Button 6 to set position") -> ()  [unwired: 14 in, 1 out]
          }
        }
      }
      frame "One_Axis_MotionMagic" {
        n160 = global read "Constants.vi" "Rotations\nTo Travel"() -> (w278:dbl)
        n161 = global read "Constants.vi" "Sensor Units\nPer Rotation"() -> (w286:i32)
        n162 = Multiply(x=w280, y=w278) -> (x*y=w287:dbl)
        n163 = Multiply(x=w287, y=w286) -> (x*y=w279:dbl)
        n164 = case shown="\"On\"" w281 {
          tunnel: w285 -> [_ w292]
          tunnel: w283 -> [_ w288]
          tunnel: w279 -> [_ w290]
          frame Default {
          }
          frame "On" {
            w291 = T15 7 items=["PercentOutput"=0, "Position"=1, "Velocity"=2, "Current"=3, "Follower"=5, "MotionProfile"=6, "MotionMagic"=7, "MotionProfileArc"=10, "Disabled"=15] ("Control Mode")
            n165 = call <vilib>:"CTRE_Phoenix_MotorControl_Set.vi"("Output"=w290, "Control Mode"=w291, "PhoenixMotorControlDevRef"=w292) -> ("PhoenixMotorControlDevRef"=w289:T2)  [unwired: 7 in, 1 out]
            n166 = call <vilib>:"CTRE_Phoenix_MotorControl_Follow.vi"("Master Controller to Follow"=w289, "PhoenixMotorControlDevRef"=w288) -> ()  [unwired: 8 in, 2 out]
          }
        }
        n167 = case shown="True" w282 {
          tunnel: w285 -> [_ w295]
          tunnel: w283 -> [_ w294]
          tunnel: w284 -> [_ w293]
          frame False {
          }
          frame True {
            n168 = call "ZeroSensors.vi"("Pigeon"=w293, "Talon 2"=w294, "Talon 1"=w295) -> ("Talon 2"=w296:T2, "Talon 1"=w297:T2)  [unwired: 6 in, 1 out]
            n169 = global read "Constants.vi" "Distance Slot"() -> (w298:i32)
            n170 = global read "Constants.vi" "PID Primary"() -> (w299:i32)
            n171 = call "Stop Motors.vi"("Talon SRX 2"=w296, "Talon SRX 1"=w297) -> ("Talon SRX 1"=w300:T2)  [unwired: 8 in, 1 out]
            n172 = call <vilib>:"CTRE_Phoenix_MotorControl_SelectProfile Slot.vi"("pidLoopIdx"=w299, "slotIdx"=w298, "PhoenixMotorControlDevRef"=w300) -> ()  [unwired: 7 in, 2 out]
            n173 = call <vilib>:"WPI_UtilitiesFRC SendMessageToConsole.vi"("Message"="One Axis Motion Magic Selected\nPress Button 6 to set position") -> ()  [unwired: 14 in, 1 out]
          }
        }
      }
      frame "One_Axis_MotionMagic_CustomFeedFwd" {
        n174 = global read "Constants.vi" "Rotations\nTo Travel"() -> (w311:dbl)
        n175 = global read "Constants.vi" "Sensor Units\nPer Rotation"() -> (w313:i32)
        n176 = Multiply(x=w304, y=0.25) -> (x*y=w302:dbl)
        n177 = Multiply(x=w310, y=w311) -> (x*y=w314:dbl)
        n178 = Multiply(x=w314, y=w313) -> (x*y=w312:dbl)
        n179 = case shown="\"On\"" w309 {
          tunnel: w305 -> [_ w321]
          tunnel: w306 -> [_ w317]
          tunnel: w312 -> [_ w319]
          tunnel: w302 -> [_ w316]
          frame Default {
          }
          frame "On" {
            w320 = T15 7 items=["PercentOutput"=0, "Position"=1, "Velocity"=2, "Current"=3, "Follower"=5, "MotionProfile"=6, "MotionMagic"=7, "MotionProfileArc"=10, "Disabled"=15] ("Control Mode")
            n180 = call <vilib>:"CTRE_Phoenix_MotorControl_Set.vi"("Demand1"=w316, "DemandType"=T11."DemandType_ArbitraryFeedForward", "Output"=w319, "Control Mode"=w320, "PhoenixMotorControlDevRef"=w321) -> ("PhoenixMotorControlDevRef"=w318:T2)  [unwired: 5 in, 1 out]
            n181 = call <vilib>:"CTRE_Phoenix_MotorControl_Follow.vi"("Master Controller to Follow"=w318, "PhoenixMotorControlDevRef"=w317) -> ()  [unwired: 8 in, 2 out]
          }
        }
        n182 = case shown="True" w308 {
          tunnel: w305 -> [_ w323]
          tunnel: w306 -> [_ w322]
          tunnel: w307 -> [_ _]
          frame False {
          }
          frame True {
            n183 = global read "Constants.vi" "Distance Slot"() -> (w324:i32)
            n184 = global read "Constants.vi" "PID Primary"() -> (w325:i32)
            n185 = call "Stop Motors.vi"("Talon SRX 2"=w322, "Talon SRX 1"=w323) -> ("Talon SRX 1"=w326:T2)  [unwired: 8 in, 1 out]
            n186 = call <vilib>:"CTRE_Phoenix_MotorControl_SelectProfile Slot.vi"("pidLoopIdx"=w325, "slotIdx"=w324, "PhoenixMotorControlDevRef"=w326) -> ()  [unwired: 7 in, 2 out]
            n187 = call <vilib>:"WPI_UtilitiesFRC SendMessageToConsole.vi"("Message"="One Axis Motion Magic with Custom Feed Fwd Selected\nPress Button 6 to set position") -> ()  [unwired: 14 in, 1 out]
          }
        }
      }
      frame "Two_Axis_MotionMagic" {
        n188 = global read "Constants.vi" "Sensor Units\nPer Rotation"() -> (w340:i32)
        n189 = global read "Constants.vi" "Turn Travel\nUnits Per Rotation"() -> (w337:dbl)
        n190 = global read "Constants.vi" "Rotations\nTo Travel"() -> (w339:dbl)
        n191 = Multiply(x=w332, y=w337) -> (x*y=w336:dbl)
        n192 = Multiply(x=w333, y=w340) -> (x*y=w341:dbl)
        n193 = Negate(x=w336) -> (-x=w335:dbl)
        n194 = Multiply(x=w341, y=w339) -> (x*y=w338:dbl)
        n195 = case shown="\"On\"" w334 {
          tunnel: w329 -> [_ w349]
          tunnel: w330 -> [_ w343]
          tunnel: w335 -> [_ w345]
          tunnel: w338 -> [_ w347]
          frame Default {
          }
          frame "On" {
            w348 = T15 7 items=["PercentOutput"=0, "Position"=1, "Velocity"=2, "Current"=3, "Follower"=5, "MotionProfile"=6, "MotionMagic"=7, "MotionProfileArc"=10, "Disabled"=15] ("Control Mode")
            n196 = call <vilib>:"CTRE_Phoenix_MotorControl_Set.vi"("Demand1"=w345, "DemandType"=T11."DemandType_AuxPID", "Output"=w347, "Control Mode"=w348, "PhoenixMotorControlDevRef"=w349) -> ("PhoenixMotorControlDevRef"=w344:T2)  [unwired: 5 in, 1 out]
            n197 = call <vilib>:"CTRE_Phoenix_MotorControl_Follow.vi"("FollowerType"=T12."FollowerType_AuxOutput1", "Master Controller to Follow"=w344, "PhoenixMotorControlDevRef"=w343) -> ()  [unwired: 7 in, 2 out]
          }
        }
        n198 = case shown="True" w328 {
          tunnel: w329 -> [_ w358]
          tunnel: w330 -> [_ w357]
          tunnel: w331 -> [_ w356]
          frame False {
          }
          frame True {
            n199 = global read "Constants.vi" "Distance Slot"() -> (w353:i32)
            n200 = global read "Constants.vi" "PID Primary"() -> (w354:i32)
            n201 = global read "Constants.vi" "Turn Slot"() -> (w352:i32)
            n202 = global read "Constants.vi" "PID Turn"() -> (w351:i32)
            n203 = call "ZeroSensors.vi"("Pigeon"=w356, "Talon 2"=w357, "Talon 1"=w358) -> ("Talon 2"=w359:T2, "Talon 1"=w360:T2)  [unwired: 6 in, 1 out]
            n204 = call "Stop Motors.vi"("Talon SRX 2"=w359, "Talon SRX 1"=w360) -> ("Talon SRX 1"=w355:T2)  [unwired: 8 in, 1 out]
            n205 = call <vilib>:"CTRE_Phoenix_MotorControl_SelectProfile Slot.vi"("pidLoopIdx"=w354, "slotIdx"=w353, "PhoenixMotorControlDevRef"=w355) -> ("PhoenixMotorControlDevRef"=w350:T2)  [unwired: 7 in, 1 out]
            n206 = call <vilib>:"CTRE_Phoenix_MotorControl_SelectProfile Slot.vi"("pidLoopIdx"=w351, "slotIdx"=w352, "PhoenixMotorControlDevRef"=w350) -> ()  [unwired: 7 in, 2 out]
            n207 = call <vilib>:"WPI_UtilitiesFRC SendMessageToConsole.vi"("Message"="Two Axis Motion Magic Selected\nPress Button 6 to set position") -> ()  [unwired: 14 in, 1 out]
          }
        }
      }
      frame "One_Axis_MotionProfile" {
        n208 = case shown="\"Off\"" w363 {
          tunnel: w366 -> [_ w368 w374 w379]
          tunnel: w365 -> [_ w373 w376 w378]
          tunnel: w362 -> [_ _ w375 _]
          frame Default {
          }
          frame "Off->On" {
            w372 = T16 6 items=["MotionProfile"=6, "MotionProfileArc"=10] ("Control Mode")
            n209 = call <vilib>:"CTRE_Phoenix_MotorControl_BufferedTrajectoryPointStream_GetDeviceReference.vi"("refnum name"="mpStream") -> ("BufferedTrajectoryPointStream_DevRef"=w369:T17)  [unwired: 9 in, 1 out]
            n210 = call <vilib>:"CTRE_Phoenix_MotorControl_StartMotionProfile.vi"("BufferedTrajectoryPointStream_DevRef"=w369, "Control Mode"=w372, "minBufferedPts"=u32 10, "PhoenixMotorControlDevRef"=w368) -> ("PhoenixMotorControlDevRef"=w367:T2)  [unwired: 6 in, 1 out]
            n211 = call <vilib>:"CTRE_Phoenix_MotorControl_Follow.vi"("Master Controller to Follow"=w367, "PhoenixMotorControlDevRef"=w373) -> ()  [unwired: 8 in, 2 out]
          }
          frame "On->Off" {
            n212 = call "ZeroSensors.vi"("Pigeon"=w375, "Talon 2"=w376, "Talon 1"=w374) -> ()  [unwired: 6 in, 3 out]
          }
          frame "Off" {
            w377 = T15 0 items=["PercentOutput"=0, "Position"=1, "Velocity"=2, "Current"=3, "Follower"=5, "MotionProfile"=6, "MotionMagic"=7, "MotionProfileArc"=10, "Disabled"=15] ("Control Mode")
            n213 = call <vilib>:"CTRE_Phoenix_MotorControl_Set.vi"("Output"=0.0, "Control Mode"=w377, "PhoenixMotorControlDevRef"=w379) -> ("PhoenixMotorControlDevRef"=w381:T2)  [unwired: 7 in, 1 out]
            n214 = call <vilib>:"CTRE_Phoenix_MotorControl_Follow.vi"("Master Controller to Follow"=w381, "PhoenixMotorControlDevRef"=w378) -> ()  [unwired: 8 in, 2 out]
          }
        }
        n215 = case shown="True" w364 {
          tunnel: w366 -> [_ w384]
          tunnel: w365 -> [_ w383]
          tunnel: w362 -> [_ w382]
          frame False {
          }
          frame True {
            n216 = call "ZeroSensors.vi"("Pigeon"=w382, "Talon 2"=w383, "Talon 1"=w384) -> ("Talon 2"=w385:T2, "Talon 1"=w386:T2)  [unwired: 6 in, 1 out]
            n217 = call "Stop Motors.vi"("Talon SRX 2"=w385, "Talon SRX 1"=w386) -> ()  [unwired: 8 in, 2 out]
            n218 = call <vilib>:"WPI_UtilitiesFRC SendMessageToConsole.vi"("Message"="One Axis Motion Profile Selected\nPress Button 6 to fire the profile") -> ()  [unwired: 14 in, 1 out]
          }
        }
      }
      frame "Two_Axis_MotionProfile" {
        n219 = case shown="\"Off->On\"" w391 {
          tunnel: w390 -> [_ w396 w401 w406]
          tunnel: w389 -> [_ w400 w403 w405]
          tunnel: w388 -> [_ _ w402 _]
          frame Default {
          }
          frame "Off->On" {
            w399 = T16 10 items=["MotionProfile"=6, "MotionProfileArc"=10] ("Control Mode")
            n220 = call <vilib>:"CTRE_Phoenix_MotorControl_BufferedTrajectoryPointStream_GetDeviceReference.vi"("refnum name"="mpTurnStream") -> ("BufferedTrajectoryPointStream_DevRef"=w397:T17)  [unwired: 9 in, 1 out]
            n221 = call <vilib>:"CTRE_Phoenix_MotorControl_StartMotionProfile.vi"("BufferedTrajectoryPointStream_DevRef"=w397, "Control Mode"=w399, "minBufferedPts"=u32 10, "PhoenixMotorControlDevRef"=w396) -> ("PhoenixMotorControlDevRef"=w395:T2)  [unwired: 6 in, 1 out]
            n222 = call <vilib>:"CTRE_Phoenix_MotorControl_Follow.vi"("FollowerType"=T12."FollowerType_AuxOutput1", "Master Controller to Follow"=w395, "PhoenixMotorControlDevRef"=w400) -> ()  [unwired: 7 in, 2 out]
          }
          frame "On->Off" {
            n223 = call "ZeroSensors.vi"("Pigeon"=w402, "Talon 2"=w403, "Talon 1"=w401) -> ()  [unwired: 6 in, 3 out]
          }
          frame "Off" {
            w404 = T15 0 items=["PercentOutput"=0, "Position"=1, "Velocity"=2, "Current"=3, "Follower"=5, "MotionProfile"=6, "MotionMagic"=7, "MotionProfileArc"=10, "Disabled"=15] ("Control Mode")
            n224 = call <vilib>:"CTRE_Phoenix_MotorControl_Set.vi"("Output"=0.0, "Control Mode"=w404, "PhoenixMotorControlDevRef"=w406) -> ("PhoenixMotorControlDevRef"=w408:T2)  [unwired: 7 in, 1 out]
            n225 = call <vilib>:"CTRE_Phoenix_MotorControl_Follow.vi"("Master Controller to Follow"=w408, "PhoenixMotorControlDevRef"=w405) -> ()  [unwired: 8 in, 2 out]
          }
        }
        n226 = case shown="True" w392 {
          tunnel: w390 -> [_ w411]
          tunnel: w389 -> [_ w410]
          tunnel: w388 -> [_ w409]
          frame False {
          }
          frame True {
            n227 = call "ZeroSensors.vi"("Pigeon"=w409, "Talon 2"=w410, "Talon 1"=w411) -> ("Talon 2"=w412:T2, "Talon 1"=w413:T2)  [unwired: 6 in, 1 out]
            n228 = call "Stop Motors.vi"("Talon SRX 2"=w412, "Talon SRX 1"=w413) -> ()  [unwired: 8 in, 2 out]
            n229 = call <vilib>:"WPI_UtilitiesFRC SendMessageToConsole.vi"("Message"="Two Axis Motion Profile Selected\nPress Button 6 to fire the profile") -> ()  [unwired: 14 in, 1 out]
          }
        }
      }
    }
  }
